vi "DCIMG to TIFF conversion_multiple files.vi"(0 "Volume number":dbl, 1 "IsSingleColor":bool, 5 "Input File Path":path, 7 "Input File Name":string, 9 "Output Path":path, 11 "error in (no error)":errorcluster, 12 "error in (no error) 2":errorcluster) -> (6 "Keys dual color":string[](array[string]), 8 "Total":i32, 10 "Index":i32, 13 "Error Out":errorcluster, 14 "Total Dual color":i32, 15 "Index Dual color":i32)   [LabVIEW 2016]
panel:
  out "Custom Data Out":string
  out "Metadata":string
  # "This is an example of how to read the images\nwithin a DCIMG file and write them to TIFF files."
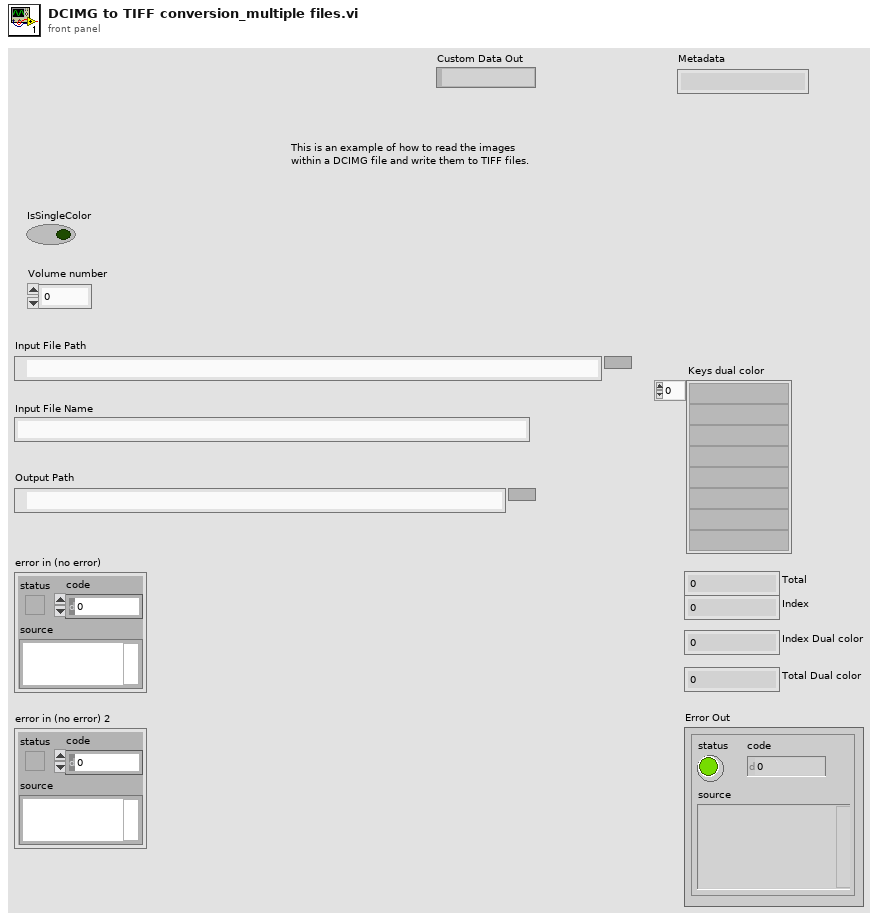
[diagram p1: front panel]
types:
  T1 = cluster{"Rows Per Strip":i32, "Photometric":i32, "Compression Type":i32}
  T2 = typedef "Image Type" = u32
  T3 = typedef "IMAQ Image.ctl" = refnum<image>
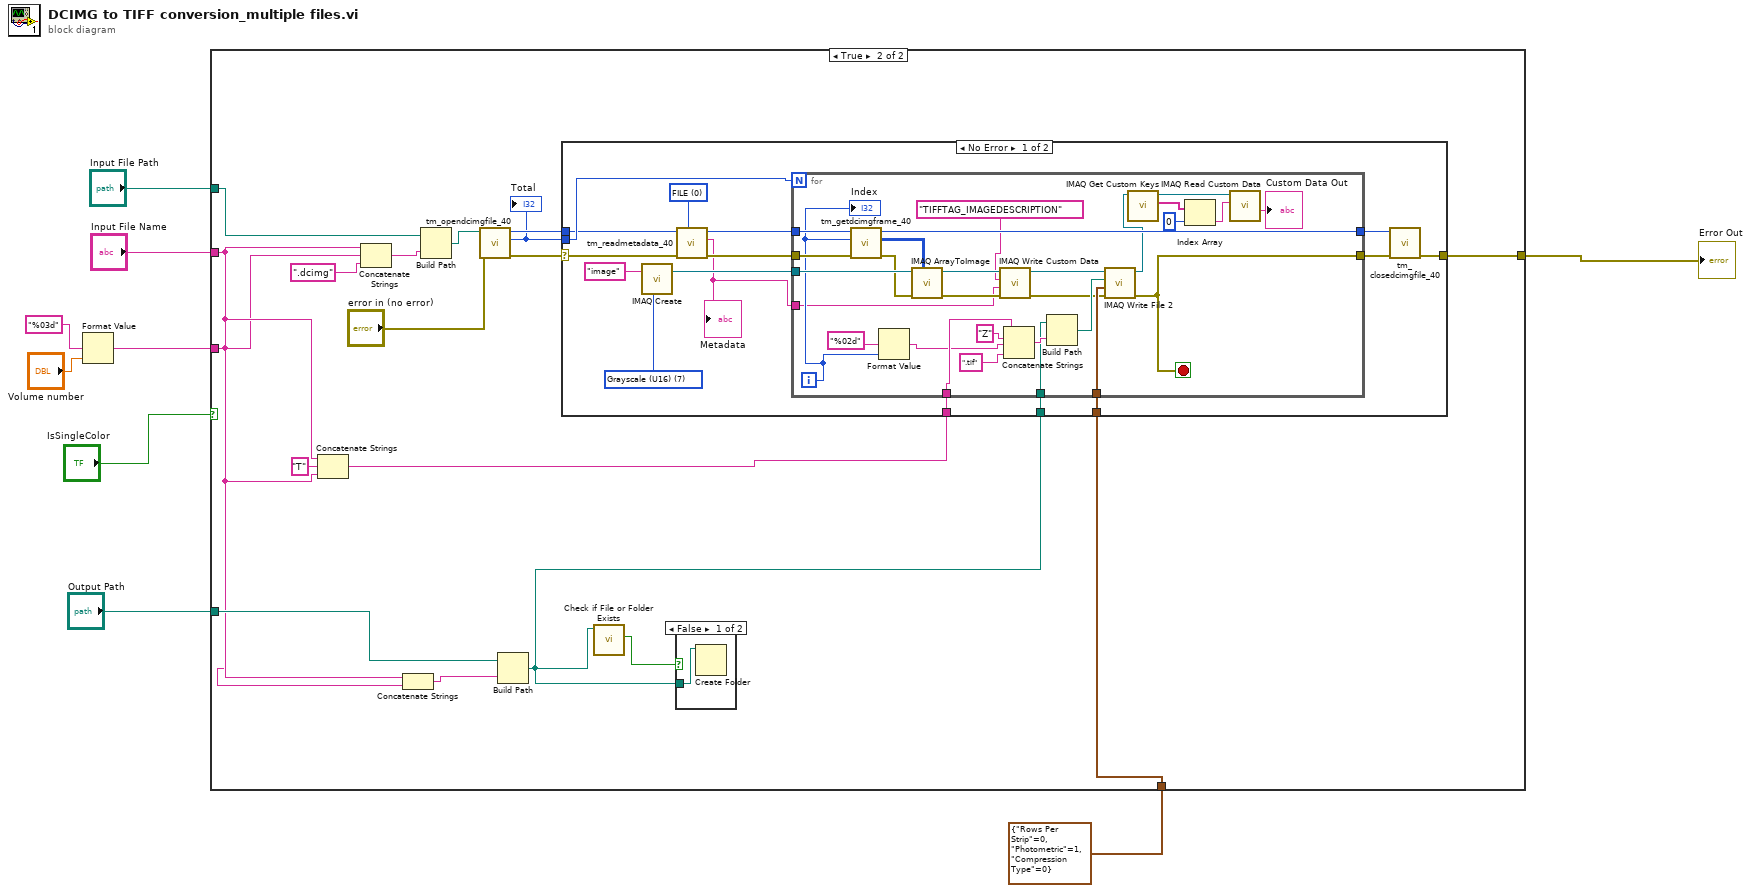
[diagram p0: block diagram]
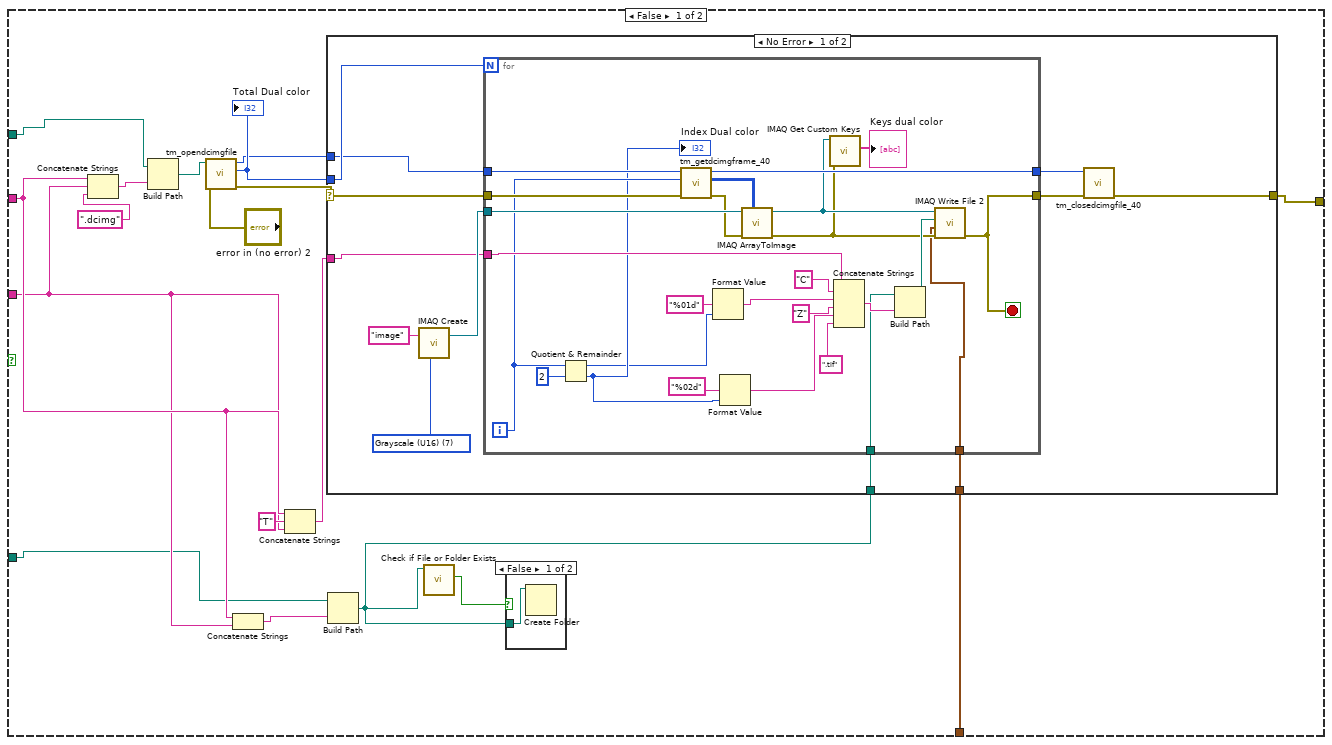
[diagram p2: hidden frame]
diagram:
  n1 = Format Value(format string="%03d", value (0)="Volume number") -> (output string=w3:string)  [unwired: 1 in]
  n2 = case shown="True" "IsSingleColor" {
    tunnel: [w11 w82] -> w9
    tunnel: "Output Path" -> [w12 w80]
    tunnel: "Input File Path" -> [w15 w76]
    tunnel: "Input File Name" -> [w14 w72]
    tunnel: w3 -> [w13 w69]
    tunnel: T1 {"Rows Per Strip"=0, "Photometric"=1, "Compression Type"=0} ("TIFF Options") -> [w10 w68]
    frame False {
      n3 = Concatenate Strings(w14, w13, ".dcimg" ("string")) -> (w25:string)
      n4 = Build Path(base path=w15, name or relative path=w25) -> (appended path=w23:path)
      n5 = call <userlib>:"tm_opendcimgfile.vi"("error in (no error)"="error in (no error) 2", "Path"=w23) -> ("error out"=w16:errorcluster, "Total Frames"=w18:i32, "File Handle"=w17:u32)  [unwired: 7 in]
      "Total Dual color" <- w18
      n6 = Concatenate Strings(w14, w13) -> (w22:string)
      n7 = Concatenate Strings(w14, "T" ("string"), w13) -> (w26:string)
      n8 = Build Path(base path=w12, name or relative path=w22) -> (appended path=w21:path)
      n9 = case shown="No Error" w16 {
        selector: w16 -> [w37 w67]
        tunnel: w17 -> [w38 _]
        tunnel: [w40 w67] -> w11
        tunnel: w18 -> [w39 _]
        tunnel: w21 -> [w31 _]
        tunnel: w26 -> [w30 _]
        tunnel: w10 -> [w29 _]
        frame No Error {
          w35 = T2 7 items=["Grayscale (U8)", "Grayscale (I16)", "Grayscale (SGL)", "Complex (CSG)", "RGB (U32)", "HSL (U32)", "RGB (U64)", "Grayscale (U16)"] ("Image Type")
          n10 = call "IMAQ Create"("Image Name"="image", "Image Type"=w35) -> ("New Image"=w34:T3)  [unwired: 3 in, 1 out]
          n11 = for {
            N: w39 -> [_]
            tunnel: w38 -> [w66]
            tunnel: w37 -> [w65]
            tunnel: w34 -> [w64]
            tunnel: [w59] -> w32
            tunnel: [w62] -> w33
            tunnel: w31 -> [w57]
            tunnel: w30 -> [w56]
            tunnel: w29 -> [w41]
            i -> [w50]
            stop <- w59 stop-if-true
            n12 = Quotient & Remainder(x=w50, y=2) -> (x-y*floor(x/y)=w44:i32, floor(x/y)=w48:i32)
            "Index Dual color" <- w48
            n13 = call <userlib>:"tm_getdcimgframe_40.vi"("error in (no error)"=w65, "Frame Index"=w50, "File Handle in"=w66) -> ("error out"=w63:errorcluster, "Data"=w60:u16[][], "File Handle out"=w62:u32)  [unwired: 5 in, 1 out]
            n14 = Format Value(format string="%01d", value (0)=w44) -> (output string=w42:string)  [unwired: 1 in]
            n15 = Format Value(format string="%02d", value (0)=w48) -> (output string=w43:string)  [unwired: 1 in]
            n16 = call "IMAQ ArrayToImage"("Image Pixels (U16)"=w60, "error in (no error)"=w63, "Image"=w64) -> ("error out"=w54:errorcluster, "Image Out"=w55:T3)  [unwired: 7 in]
            n17 = call "IMAQ Get Custom Keys"("error in (no error)"=w54, "Image"=w55) -> ("Keys"=→"Keys dual color":string[])  [unwired: 6 in, 3 out]
            n18 = Concatenate Strings(w56, "C" ("string"), w42, "Z" ("string"), w43, ".tif" ("regular expression (\"\")")) -> (w61:string)
            n19 = Build Path(base path=w57, name or relative path=w61) -> (appended path=w58:path)
            n20 = call-poly "IMAQ Write File 2"("error in (no error)"=w54, "TIFF Options"=w41, "File Path"=w58, "Image"=w55) -> ("error out"=w59:errorcluster)  [unwired: 6 in, 1 out]
          }
          n21 = call <userlib>:"tm_closedcimgfile_40.vi"("error in (no error)"=w32, "File Handle"=w33) -> ("error out"=w40:errorcluster)  [unwired: 9 in]
        }
        frame Error {
        }
      }
      n22 = call <vilib>:"Check if File or Folder Exists.vi"("path"=w21) -> ("file or folder exists?"=w20:bool)  [unwired: 8 in, 2 out]
      n23 = case shown="False" w20 {
        tunnel: w21 -> [w28 _]
        frame False {
          n24 = Create Folder(path (use dialog)=w28) -> ()  [unwired: 2 in, 3 out]
        }
        frame True {
        }
      }
    }
    frame True {
      n25 = Concatenate Strings(w72, "T" ("string"), w69) -> (w71:string)
      n26 = Concatenate Strings(w72, w69, ".dcimg" ("string")) -> (w73:string)
      n27 = Concatenate Strings(w72, w69) -> (w77:string)
      n28 = Build Path(base path=w76, name or relative path=w73) -> (appended path=w75:path)
      n29 = call <userlib>:"tm_opendcimgfile_40.vi"("error in (no error)"="error in (no error)", "Path"=w75) -> ("error out"=w85:errorcluster, "Total Frames"=w83:i32, "File Handle"=w84:u32)  [unwired: 7 in]
      "Total" <- w83
      n30 = Build Path(base path=w80, name or relative path=w77) -> (appended path=w78:path)
      n31 = case shown="No Error" w85 {
        selector: w85 -> [w90 w132]
        tunnel: w84 -> [w92 _]
        tunnel: [w102 w132] -> w82
        tunnel: w83 -> [w101 _]
        tunnel: w78 -> [w95 _]
        tunnel: w71 -> [w94 _]
        tunnel: w68 -> [w93 _]
        frame No Error {
          w88 = 0 items=["FILE"=0, "FRAME"=2] ("Type")
          w99 = T2 7 items=["Grayscale (U8)", "Grayscale (I16)", "Grayscale (SGL)", "Complex (CSG)", "RGB (U32)", "HSL (U32)", "RGB (U64)", "Grayscale (U16)"] ("Image Type")
          n32 = call "IMAQ Create"("Image Name"="image", "Image Type"=w99) -> ("New Image"=w98:T3)  [unwired: 3 in, 1 out]
          n33 = call <userlib>:"tm_readmetadata_40.vi"("Type"=w88, "error in (no error)"=w90, "File Handle"=w92) -> ("error out"=w89:errorcluster, "Metadata"=w87:string, "File Handle"=w91:u32)  [unwired: 6 in]
          "Metadata" <- w87
          n34 = for {
            N: w101 -> [_]
            tunnel: w91 -> [w131]
            tunnel: w89 -> [w130]
            tunnel: w98 -> [w129]
            tunnel: [w124] -> w96
            tunnel: [w127] -> w97
            tunnel: w95 -> [w122]
            tunnel: w94 -> [w121]
            tunnel: w93 -> [w113]
            tunnel: w87 -> [w110]
            i -> [w115]
            stop <- w124 stop-if-true
            n35 = call <userlib>:"tm_getdcimgframe_40.vi"("error in (no error)"=w130, "Frame Index"=w115, "File Handle in"=w131) -> ("error out"=w128:errorcluster, "Data"=w125:u16[][], "File Handle out"=w127:u32)  [unwired: 5 in, 1 out]
            n36 = Format Value(format string="%02d", value (0)=w115) -> (output string=w116:string)  [unwired: 1 in]
            n37 = call "IMAQ ArrayToImage"("Image Pixels (U16)"=w125, "error in (no error)"=w128, "Image"=w129) -> ("error out"=w119:errorcluster, "Image Out"=w120:T3)  [unwired: 7 in]
            n38 = call "IMAQ Write Custom Data"("error in (no error)"=w119, "Custom Data In"=w110, "Key"="TIFFTAG_IMAGEDESCRIPTION", "Image"=w120) -> ("error out"=w111:errorcluster, "Image Out"=w112:T3)  [unwired: 6 in]
            n39 = Concatenate Strings(w121, "Z" ("string"), w116, ".tif" ("regular expression (\"\")")) -> (w126:string)
            n40 = Build Path(base path=w122, name or relative path=w126) -> (appended path=w123:path)
            n41 = call-poly "IMAQ Write File 2"("error in (no error)"=w111, "TIFF Options"=w113, "File Path"=w123, "Image"=w112) -> ("error out"=w124:errorcluster, "Image Out (duplicate)"=w108:T3)  [unwired: 6 in]
            n42 = call "IMAQ Get Custom Keys"("Image"=w108) -> ("Keys"=w106:string[], "Image (duplicate)"=w107:T3)  [unwired: 7 in, 2 out]
            n43 = Index Array(array=w106, index=0) -> (element=w104:string)
            n44 = call "IMAQ Read Custom Data"("Key"=w104, "Image"=w107) -> ("Custom Data Out"=→"Custom Data Out":string)  [unwired: 7 in, 2 out]
            "Index" <- w115
          }
          n45 = call <userlib>:"tm_closedcimgfile_40.vi"("error in (no error)"=w96, "File Handle"=w97) -> ("error out"=w102:errorcluster)  [unwired: 9 in]
        }
        frame Error {
        }
      }
      n46 = call <vilib>:"Check if File or Folder Exists.vi"("path"=w78) -> ("file or folder exists?"=w79:bool)  [unwired: 8 in, 2 out]
      n47 = case shown="False" w79 {
        tunnel: w78 -> [w86 _]
        frame False {
          n48 = Create Folder(path (use dialog)=w86) -> ()  [unwired: 2 in, 3 out]
        }
        frame True {
        }
      }
    }
  }
  "Error Out" <- w9
